vi "BRig_dataMTrig_warmup_cNoLick_L_reset.vi"() -> (2 "output_warmup_cNoLick_L_reset":i32)   [LabVIEW 2014]
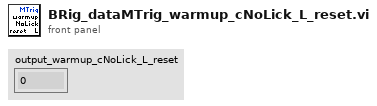
[diagram p1: front panel]
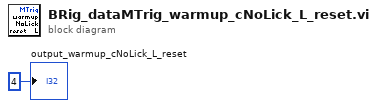
[diagram p0: block diagram]
diagram:
  "output_warmup_cNoLick_L_reset" <- 4 ("output_iBlock")
